vi "Generate Date Folder.vi"(11 "root dir":path=path "C:/Users/Labmember/Desktop/NoiseData") -> (3 "today's folder":path)   [LabVIEW 2015]
panel:
  out "date/time string":string
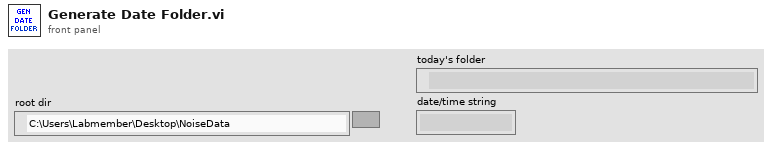
[diagram p1: front panel]
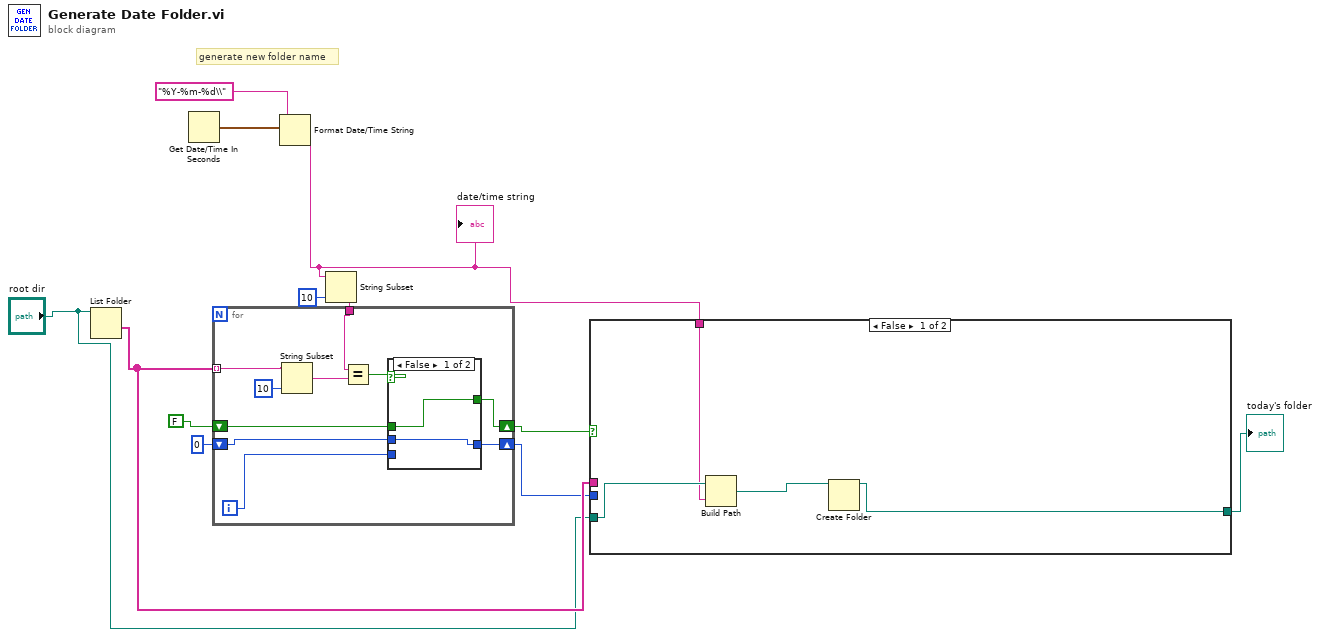
[diagram p0: block diagram]
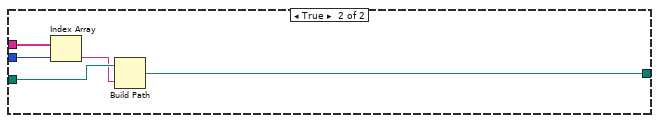
[diagram p2: hidden frame]
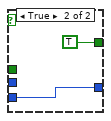
[diagram p3: hidden frame]
diagram:
  # "generate new folder name"
  n1 = List Folder(path="root dir") -> (folder names=w6:string[])  [unwired: 3 in, 3 out]
  n2 = Get Date/Time In Seconds() -> (seconds since 1Jan1904=w11:timestamp)
  n3 = Format Date/Time String(time format string (%c)="%Y-%m-%d\\", seconds (now)=w11) -> (date/time string=w1:string)  [unwired: 1 in]
  "date/time string" <- w1
  n4 = String Subset(string=w1, length (rest)=10 ("length (rest)")) -> (substring=w9:string)  [unwired: 1 in]
  n5 = for {
    tunnel: w6 -> [w22] mode=indexing
    tunnel: w9 -> [w19]
    shift-right: [w17] -> w5
    shift-left: FALSE ("x = y?") -> [w16]
    shift-right: [w14] -> w4
    shift-left: 0 -> [w13]
    i -> [w15]
    n6 = String Subset(string=w22, length (rest)=10 ("length (rest)")) -> (substring=w20:string)  [unwired: 1 in]
    n7 = Equal?(x=w19, y=w20) -> (x = y?=w18:bool)
    n8 = case shown="False" w18 {
      tunnel: [w24 TRUE ("x = y?")] -> w17
      tunnel: w16 -> [w24 _]
      tunnel: w15 -> [_ w25]
      tunnel: [w23 w25] -> w14
      tunnel: w13 -> [w23 _]
      frame False {
      }
      frame True {
      }
    }
  }
  n9 = case shown="False" w5 {
    tunnel: w6 -> [_ w35]
    tunnel: w4 -> [_ w34]
    tunnel: "root dir" -> [w30 w33]
    tunnel: [w27 w31] -> w2
    tunnel: w1 -> [w29 _]
    frame False {
      n10 = Build Path(base path=w30, name or relative path=w29) -> (appended path=w28:path)
      n11 = Create Folder(path (use dialog)=w28) -> (created path=w27:path)  [unwired: 2 in, 2 out]
    }
    frame True {
      n12 = Index Array(array=w35, index=w34) -> (element=w32:string)
      n13 = Build Path(base path=w33, name or relative path=w32) -> (appended path=w31:path)
    }
  }
  "today's folder" <- w2
